vi "Create StringArrayMsg.vi"(8 "error in (no error)":errorcluster, 10 "Message Data":string[](array[string]), 11 "Message Name":string) -> (0 "error out":errorcluster, 3 "StringArrayMsg out":refnum<class "StringArrayMsg.lvclass">)   [LabVIEW 2009, in "LapDog.Messaging.v2.NativeArrays.lvlib" / "StringArrayMsg.lvclass"]
doc: "Returns a StringArrayMsg object with the given name.\n\nThis method executes regardless of the error in state."
uses:
  StringArrayMsg.lvclass
  StringArrayMsg.lvclass/StringArrayMsg.ctl
  Messaging.v2/MessageObject/Message.lvclass
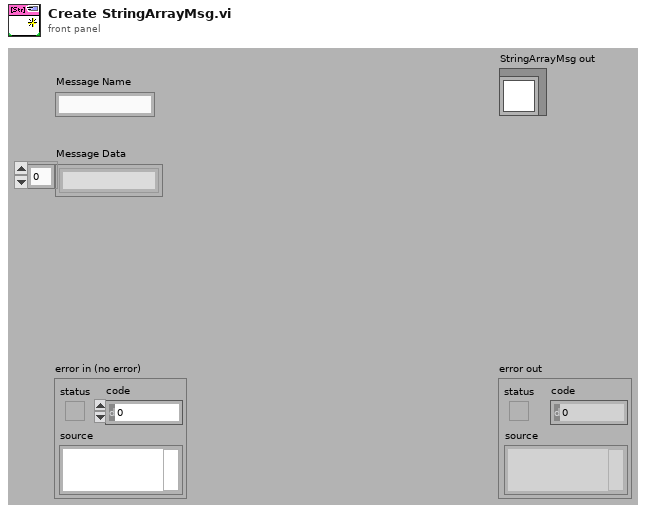
[diagram p1: front panel]
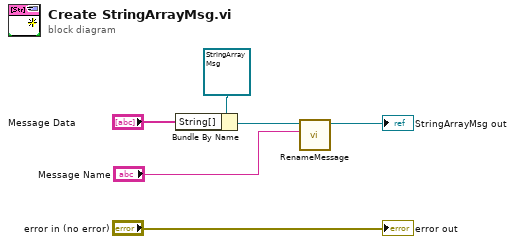
[diagram p0: block diagram]
diagram:
  n1 = Bundle By Name(cluster=refnum<class "StringArrayMsg.lvclass"> refnum ("StringMsg in"), "String[]"="Message Data") -> (w4:refnum<class "StringArrayMsg.lvclass">)
  n2 = call "RenameMessage.vi"("Message Name"="Message Name", "Message in"=w4) -> ("Message out"=→"StringArrayMsg out":refnum<class "StringArrayMsg.lvclass">)  [unwired: 8 in, 1 out]
  "error out" <- "error in (no error)"
